vi "Find Node by Comment.vi"(8 "error in (no error)":errorcluster, 10 "Node Array":refnum<k20>[](array[refnum]), 11 "Comment":string) -> (0 "error out":errorcluster, 3 "Node out":refnum<k20>)   [LabVIEW 2013]
uses:
  <vilib>/xml/Close Reference(Node).vi
  <vilib>/xml/NI_XML.lvlib
panel:
  out "Exists":bool
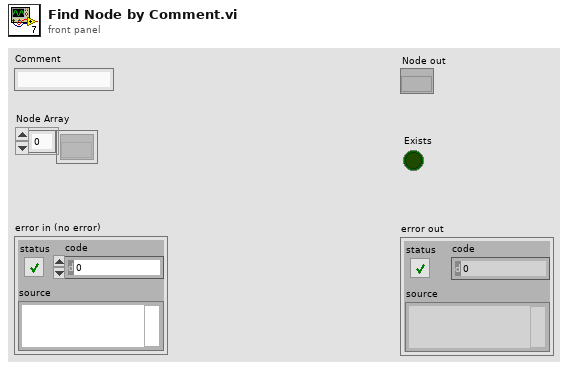
[diagram p1: front panel]
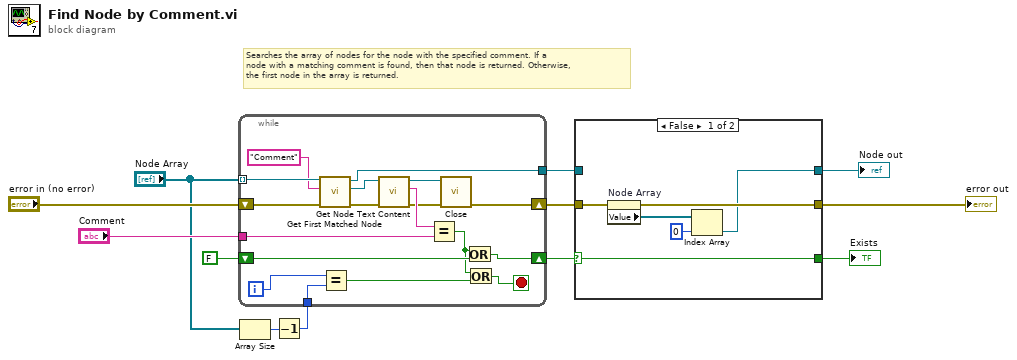
[diagram p0: block diagram]
diagram:
  # "Searches the array of nodes for the node with the specified comment. If a\nnode with a matching comment is found, then that node is returned. Otherwise,\nthe first node in the array is returned."
  n1 = Array Size(array="Node Array") -> (size(s)=w2:i32)
  n2 = Decrement(x=w2) -> (x-1=w1:i32)
  n3 = while {
    tunnel: "Node Array" -> [w30] mode=indexing
    shift-right: [w21] -> w8
    shift-left: "error in (no error)" -> [w29]
    tunnel: "Comment" -> [w24]
    tunnel: [w23] -> w7
    shift-right: [w18] -> w9
    shift-left: FALSE -> [w19]
    tunnel: w1 -> [w17]
    i -> [w16]
    stop <- w13 stop-if-true
    n4 = call <vilib>:"Get First Matched Node.vi"("error in (no error)"=w29, "XPath expression"="Comment", "node in"=w30) -> ("error out"=w28:errorcluster, "node result"=w26:refnum<k20>, "node out"=w23:refnum<k20>)  [unwired: 6 in]
    n5 = Equal?(x=w16, y=w17) -> (x = y?=w15:bool)
    n6 = call <vilib>:"Get Node Text Content.vi"("error in (no error)"=w28, "node in"=w26) -> ("error out"=w22:errorcluster, "node text"=w25:string, "node out"=w20:refnum<k20>)  [unwired: 7 in]
    n7 = Equal?(x=w25, y=w24) -> (x = y?=w14:bool)
    n8 = call-poly <vilib>:"Close.vi"("error in (no error)"=w22, "node"=w20) -> ("error out"=w21:errorcluster)  [unwired: 7 in]
    n9 = Or(x=w14, y=w19) -> (x .or. y?=w18:bool)
    n10 = Or(x=w14, y=w15) -> (x .or. y?=w13:bool)
  }
  n11 = case shown="False" w9 {
    selector: w9 -> [w31 w37]
    tunnel: w8 -> [w36 w38]
    tunnel: w7 -> [_ w39]
    tunnel: [w32 w39] -> w6
    tunnel: [w33 w38] -> w5
    tunnel: [w31 w37] -> w4
    frame False {
      n12 = property on="Node Array" class="Arr (strict)"(error in=w36) -> (error out=w33:errorcluster, "Value"=w35:refnum<k20>[])  [unwired: 1 in, 1 out]
      n13 = Index Array(array=w35, index=0) -> (element=w32:refnum<k20>)
    }
    frame True {
    }
  }
  "error out" <- w5
  "Exists" <- w4
  "Node out" <- w6
